vi "GDFreadVariableHeaders.vi"(8 "error in":errorcluster, 11 "GDFv1.x.lvclass in":refnum<class "GDFv1.x.lvclass">) -> (0 "error out":errorcluster, 2 "GDFHeader2 out":T1, 3 "GDFv1.x.lvclass out":refnum<class "GDFv1.x.lvclass">)   [LabVIEW 2016, in "GDF File Reader.lvlib" / "GDFv1.x.lvclass"]
uses:
  GDFv1.x.lvclass
  GdfHeader2.ctl
  GDFv1.x.lvclass/GDFv1.x.ctl
  GDF File Reader.lvlib
panel:
  # "This VI is a part of BCI Design library, http://www.ru-bci.org \nCopyright © 2020, Sotnikov Peter, All rights reserved. License: GNU GPLv3"
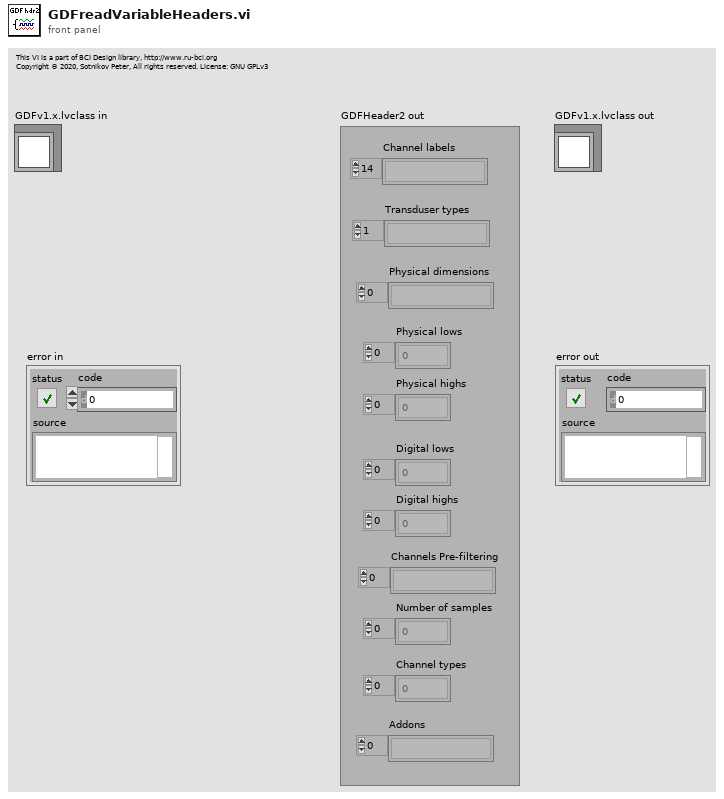
[diagram p1: front panel]
types:
  T1 = typedef "GDF File Reader.lvlib/GdfHeader2.ctl" = cluster{"Channel labels":string[], "Transduser types":string[], "Physical dimensions":string[], "Physical lows":dbl[], "Physical highs":dbl[], "Digital lows":dbl[], "Digital highs":dbl[], "Channels Pre-filtering":string[], "Number of samples":u32[], "Channel types":u32[], "Addons":string[]}
  T2 = typedef "GDF File Reader.lvlib/GdfHeader1.ctl" = cluster{"Version identificator":string, "Patient identificator":string, "Recording identificator":string, "StartDateTime":timestamp, "Header record length":i64, "Equipment Provider":u64, "Laboratory":u64, "Technician":u64, "Number of data records":i64, "Duration of a data record":cluster{"Numerator":u32, "Denominator":u32}, "Number of signals":u32}
  T3 = enum16{"big-endian, network order", "native, host order", "little-endian"}
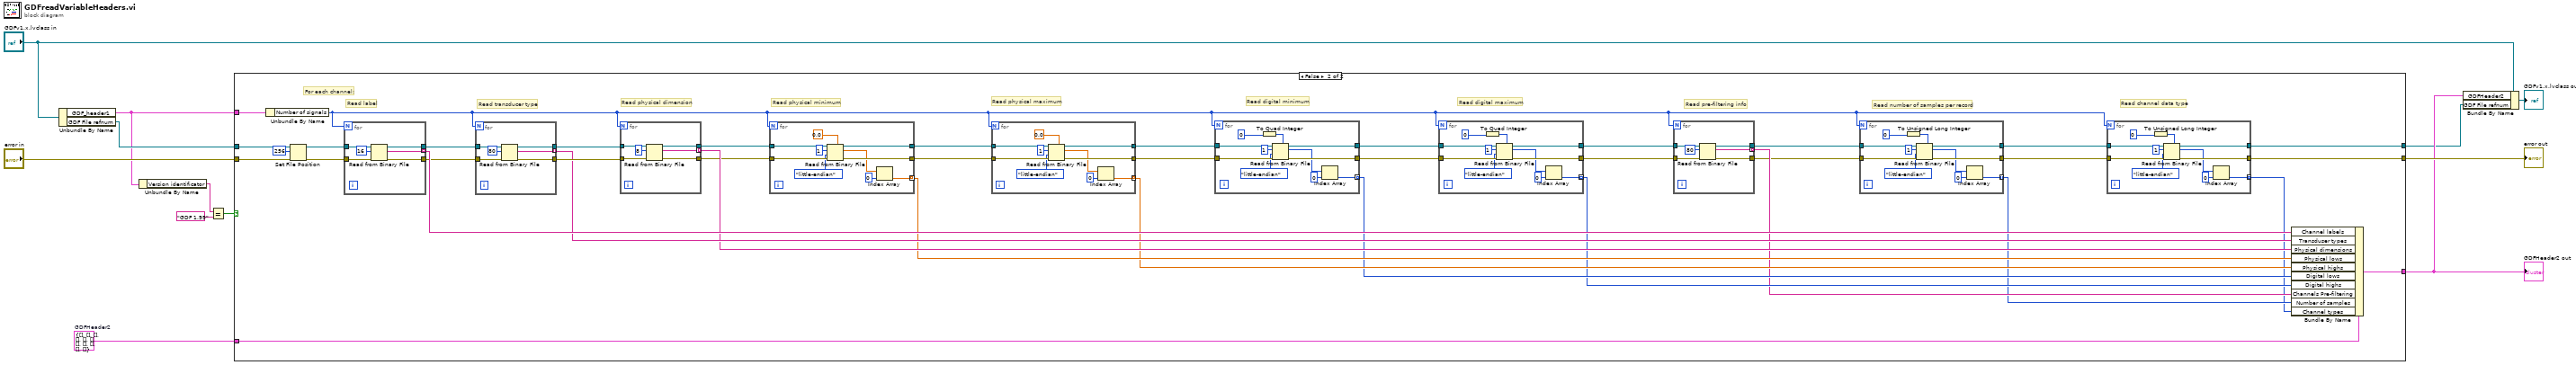
[diagram p0: block diagram]
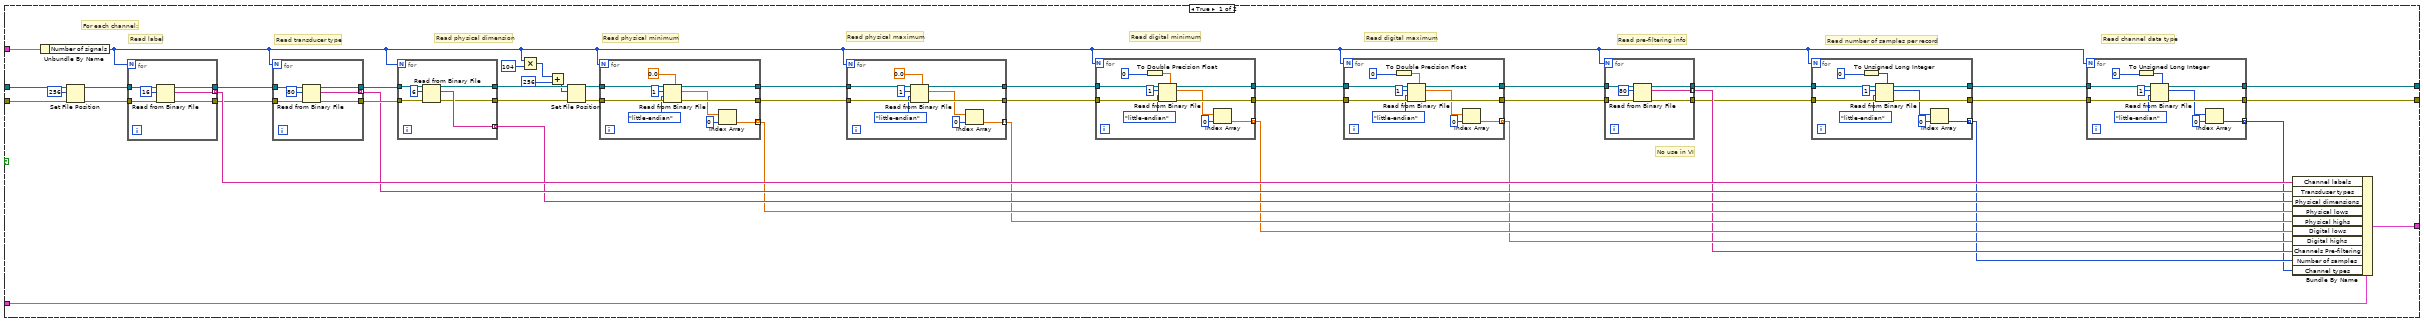
[diagram p2: hidden frame]
diagram:
  w12 = T1 {"Channel labels"=[], "Transduser types"=[], "Physical dimensions"=[], "Physical lows"=[], "Physical highs"=[], "Digital lows"=[], "Digital highs"=[], "Channels Pre-filtering"=[], "Number of samples"=[], "Channel types"=[], "Addons"=[]}  # GDFHeader2
  n1 = Unbundle By Name("GDFv1.x.lvclass in") -> ("GDF_header1"=w4:T2, "GDF File refnum"=w9:refnum<file>)
  n2 = Unbundle By Name(w4) -> ("Version identificator"=w2:string)
  n3 = Equal?(x=w2, y="GDF 1.99") -> (x = y?=w3:bool)
  n4 = case shown="False" w3 {
    tunnel: w12 -> [w57 w184]
    tunnel: "error in" -> [w56 w183]
    tunnel: [w26 w151] -> w10
    tunnel: w9 -> [w25 w149]
    tunnel: w4 -> [w24 w148]
    tunnel: [w23 w147] -> w7
    tunnel: [w22 w146] -> w6
    frame True {
      # "No use in VI"
      # "Read pre-filtering info"
      # "Read channel data type"
      # "Read number of samples per record"
      # "Read digital maximum"
      # "Read digital minimum"
      # "Read physical maximum"
      # "Read physical minimum"
      # "Read physical dimension"
      # "Read transducer type"
      # "Read label"
      # "For each channel:"
      n5 = Unbundle By Name(w24) -> ("Number of signals"=w17:u32)
      n6 = Set File Position(offset (in bytes) (0)=i64 256, refnum=w25, error in=w56) -> (refnum out=w53:refnum<file>, error out=w54:errorcluster)  [unwired: 1 in]
      n7 = for {
        N: w17 -> [_]
        tunnel: w54 -> [w145]
        tunnel: w53 -> [w144]
        tunnel: [w142] -> w50
        tunnel: [w141] -> w51
        tunnel: [w140] -> w52 mode=indexing
        n8 = Read from Binary File(8:w145, 10:16 ("count (1)"), 11:w144) -> (0:w141:errorcluster, 2:w140:string, 3:w142:refnum<file>)  [unwired: 3 in, 1 out]
      }
      n9 = for {
        N: w17 -> [_]
        tunnel: w51 -> [w139]
        tunnel: w50 -> [w138]
        tunnel: [w136] -> w48
        tunnel: [w135] -> w49
        tunnel: [w134] -> w47 mode=indexing
        n10 = Read from Binary File(8:w139, 10:80 ("count (1)"), 11:w138) -> (0:w135:errorcluster, 2:w134:string, 3:w136:refnum<file>)  [unwired: 3 in, 1 out]
      }
      n11 = for {
        N: w17 -> [_]
        tunnel: w49 -> [w133]
        tunnel: w48 -> [w132]
        tunnel: [w128] -> w20
        tunnel: [w129] -> w21
        tunnel: [w130] -> w46 mode=indexing
        n12 = Read from Binary File(8:w133, 10:6 ("count (1)"), 11:w132) -> (0:w129:errorcluster, 2:w130:string, 3:w128:refnum<file>)  [unwired: 3 in, 1 out]
      }
      n13 = Multiply(x=w17, y=u32 104) -> (x*y=w15:u32)
      n14 = Add(x=w15, y=u32 256) -> (x+y=w13:u32)
      n15 = Set File Position(offset (in bytes) (0)=w13, refnum=w20, error in=w21) -> (refnum out=w19:refnum<file>, error out=w18:errorcluster)  [unwired: 1 in]
      n16 = for {
        N: w17 -> [_]
        tunnel: w18 -> [w127]
        tunnel: w19 -> [w126]
        tunnel: [w124] -> w44
        tunnel: [w123] -> w45
        tunnel: [w118] -> w43 mode=indexing
        n17 = Read from Binary File(5:0.0, 8:w127, 9:T3."little-endian" ("byte order (0:big-endian, network order)"), 10:1 ("count (1)"), 11:w126) -> (0:w123:errorcluster, 2:w120:dbl[], 3:w124:refnum<file>)  [unwired: 1 in, 1 out]
        n18 = Index Array(array=w120, index=0) -> (element=w118:dbl)
      }
      n19 = for {
        N: w17 -> [_]
        tunnel: w45 -> [w117]
        tunnel: w44 -> [w116]
        tunnel: [w114] -> w41
        tunnel: [w113] -> w40
        tunnel: [w108] -> w42 mode=indexing
        n20 = Read from Binary File(5:0.0, 8:w117, 9:T3."little-endian" ("byte order (0:big-endian, network order)"), 10:1 ("count (1)"), 11:w116) -> (0:w113:errorcluster, 2:w110:dbl[], 3:w114:refnum<file>)  [unwired: 1 in, 1 out]
        n21 = Index Array(array=w110, index=0) -> (element=w108:dbl)
      }
      n22 = for {
        N: w17 -> [_]
        tunnel: w40 -> [w107]
        tunnel: w41 -> [w106]
        tunnel: [w105] -> w39
        tunnel: [w104] -> w38
        tunnel: [w100] -> w37 mode=indexing
        n23 = To Double Precision Float(number=0 ("count (1)")) -> (double precision float=w97:dbl)
        n24 = Read from Binary File(5:w97, 8:w107, 9:T3."little-endian" ("byte order (0:big-endian, network order)"), 10:1 ("count (1)"), 11:w106) -> (0:w104:errorcluster, 2:w102:dbl[], 3:w105:refnum<file>)  [unwired: 1 in, 1 out]
        n25 = Index Array(array=w102, index=0) -> (element=w100:dbl)
      }
      n26 = for {
        N: w17 -> [_]
        tunnel: w38 -> [w96]
        tunnel: w39 -> [w95]
        tunnel: [w94] -> w34
        tunnel: [w93] -> w35
        tunnel: [w89] -> w36 mode=indexing
        n27 = To Double Precision Float(number=0 ("count (1)")) -> (double precision float=w86:dbl)
        n28 = Read from Binary File(5:w86, 8:w96, 9:T3."little-endian" ("byte order (0:big-endian, network order)"), 10:1 ("count (1)"), 11:w95) -> (0:w93:errorcluster, 2:w91:dbl[], 3:w94:refnum<file>)  [unwired: 1 in, 1 out]
        n29 = Index Array(array=w91, index=0) -> (element=w89:dbl)
      }
      n30 = for {
        N: w17 -> [_]
        tunnel: w35 -> [w85]
        tunnel: w34 -> [w84]
        tunnel: [w82] -> w31
        tunnel: [w81] -> w32
        tunnel: [w80] -> w33 mode=indexing
        n31 = Read from Binary File(8:w85, 10:80 ("count (1)"), 11:w84) -> (0:w81:errorcluster, 2:w80:string, 3:w82:refnum<file>)  [unwired: 3 in, 1 out]
      }
      n32 = for {
        N: w17 -> [_]
        tunnel: w32 -> [w79]
        tunnel: w31 -> [w78]
        tunnel: [w77] -> w29
        tunnel: [w76] -> w30
        tunnel: [w72] -> w28 mode=indexing
        n33 = To Unsigned Long Integer(number=0 ("count (1)")) -> (unsigned 32bit integer=w69:u32)
        n34 = Read from Binary File(5:w69, 8:w79, 9:T3."little-endian" ("byte order (0:big-endian, network order)"), 10:1 ("count (1)"), 11:w78) -> (0:w76:errorcluster, 2:w74:u32[], 3:w77:refnum<file>)  [unwired: 1 in, 1 out]
        n35 = Index Array(array=w74, index=0) -> (element=w72:u32)
      }
      n36 = for {
        N: w17 -> [_]
        tunnel: w30 -> [w68]
        tunnel: w29 -> [w67]
        tunnel: [w66] -> w22
        tunnel: [w65] -> w26
        tunnel: [w61] -> w27 mode=indexing
        n37 = To Unsigned Long Integer(number=0 ("count (1)")) -> (unsigned 32bit integer=w58:u32)
        n38 = Read from Binary File(5:w58, 8:w68, 9:T3."little-endian" ("byte order (0:big-endian, network order)"), 10:1 ("count (1)"), 11:w67) -> (0:w65:errorcluster, 2:w63:u32[], 3:w66:refnum<file>)  [unwired: 1 in, 1 out]
        n39 = Index Array(array=w63, index=0) -> (element=w61:u32)
      }
      n40 = Bundle By Name(cluster=w57, "Channel labels"=w52, "Transduser types"=w47, "Physical dimensions"=w46, "Physical lows"=w43, "Physical highs"=w42, "Digital lows"=w37, "Digital highs"=w36, "Channels Pre-filtering"=w33, "Number of samples"=w28, "Channel types"=w27) -> (w23:T1)
    }
    frame False {
      # "Read pre-filtering info"
      # "Read channel data type"
      # "Read number of samples per record"
      # "Read digital maximum"
      # "Read digital minimum"
      # "Read physical maximum"
      # "Read physical minimum"
      # "Read physical dimension"
      # "Read transducer type"
      # "Read label"
      # "For each channel:"
      n41 = Unbundle By Name(w148) -> ("Number of signals"=w150:u32)
      n42 = Set File Position(offset (in bytes) (0)=i64 256, refnum=w149, error in=w183) -> (refnum out=w180:refnum<file>, error out=w181:errorcluster)  [unwired: 1 in]
      n43 = for {
        N: w150 -> [_]
        tunnel: w181 -> [w272]
        tunnel: w180 -> [w271]
        tunnel: [w269] -> w177
        tunnel: [w268] -> w178
        tunnel: [w267] -> w179 mode=indexing
        n44 = Read from Binary File(8:w272, 10:16 ("count (1)"), 11:w271) -> (0:w268:errorcluster, 2:w267:string, 3:w269:refnum<file>)  [unwired: 3 in, 1 out]
      }
      n45 = for {
        N: w150 -> [_]
        tunnel: w178 -> [w266]
        tunnel: w177 -> [w265]
        tunnel: [w263] -> w175
        tunnel: [w262] -> w176
        tunnel: [w261] -> w174 mode=indexing
        n46 = Read from Binary File(8:w266, 10:80 ("count (1)"), 11:w265) -> (0:w262:errorcluster, 2:w261:string, 3:w263:refnum<file>)  [unwired: 3 in, 1 out]
      }
      n47 = for {
        N: w150 -> [_]
        tunnel: w176 -> [w260]
        tunnel: w175 -> [w259]
        tunnel: [w257] -> w172
        tunnel: [w256] -> w171
        tunnel: [w255] -> w173 mode=indexing
        n48 = Read from Binary File(8:w260, 10:8 ("count (1)"), 11:w259) -> (0:w256:errorcluster, 2:w255:string, 3:w257:refnum<file>)  [unwired: 3 in, 1 out]
      }
      n49 = for {
        N: w150 -> [_]
        tunnel: w171 -> [w254]
        tunnel: w172 -> [w253]
        tunnel: [w251] -> w169
        tunnel: [w250] -> w170
        tunnel: [w245] -> w168 mode=indexing
        n50 = Read from Binary File(5:0.0, 8:w254, 9:T3."little-endian" ("byte order (0:big-endian, network order)"), 10:1 ("count (1)"), 11:w253) -> (0:w250:errorcluster, 2:w247:dbl[], 3:w251:refnum<file>)  [unwired: 1 in, 1 out]
        n51 = Index Array(array=w247, index=0) -> (element=w245:dbl)
      }
      n52 = for {
        N: w150 -> [_]
        tunnel: w170 -> [w244]
        tunnel: w169 -> [w243]
        tunnel: [w241] -> w166
        tunnel: [w240] -> w165
        tunnel: [w235] -> w167 mode=indexing
        n53 = Read from Binary File(5:0.0, 8:w244, 9:T3."little-endian" ("byte order (0:big-endian, network order)"), 10:1 ("count (1)"), 11:w243) -> (0:w240:errorcluster, 2:w237:dbl[], 3:w241:refnum<file>)  [unwired: 1 in, 1 out]
        n54 = Index Array(array=w237, index=0) -> (element=w235:dbl)
      }
      n55 = for {
        N: w150 -> [_]
        tunnel: w165 -> [w234]
        tunnel: w166 -> [w233]
        tunnel: [w232] -> w164
        tunnel: [w231] -> w163
        tunnel: [w227] -> w162 mode=indexing
        n56 = To Quad Integer(1:0 ("count (1)")) -> (0:w224:i64)
        n57 = Read from Binary File(5:w224, 8:w234, 9:T3."little-endian" ("byte order (0:big-endian, network order)"), 10:1 ("count (1)"), 11:w233) -> (0:w231:errorcluster, 2:w229:i64[], 3:w232:refnum<file>)  [unwired: 1 in, 1 out]
        n58 = Index Array(array=w229, index=0) -> (element=w227:i64)
      }
      n59 = for {
        N: w150 -> [_]
        tunnel: w163 -> [w223]
        tunnel: w164 -> [w222]
        tunnel: [w221] -> w159
        tunnel: [w220] -> w160
        tunnel: [w216] -> w161 mode=indexing
        n60 = To Quad Integer(1:0 ("count (1)")) -> (0:w213:i64)
        n61 = Read from Binary File(5:w213, 8:w223, 9:T3."little-endian" ("byte order (0:big-endian, network order)"), 10:1 ("count (1)"), 11:w222) -> (0:w220:errorcluster, 2:w218:i64[], 3:w221:refnum<file>)  [unwired: 1 in, 1 out]
        n62 = Index Array(array=w218, index=0) -> (element=w216:i64)
      }
      n63 = for {
        N: w150 -> [_]
        tunnel: w160 -> [w212]
        tunnel: w159 -> [w211]
        tunnel: [w209] -> w156
        tunnel: [w208] -> w157
        tunnel: [w207] -> w158 mode=indexing
        n64 = Read from Binary File(8:w212, 10:80 ("count (1)"), 11:w211) -> (0:w208:errorcluster, 2:w207:string, 3:w209:refnum<file>)  [unwired: 3 in, 1 out]
      }
      n65 = for {
        N: w150 -> [_]
        tunnel: w157 -> [w206]
        tunnel: w156 -> [w205]
        tunnel: [w204] -> w154
        tunnel: [w203] -> w155
        tunnel: [w199] -> w153 mode=indexing
        n66 = To Unsigned Long Integer(number=0 ("count (1)")) -> (unsigned 32bit integer=w196:u32)
        n67 = Read from Binary File(5:w196, 8:w206, 9:T3."little-endian" ("byte order (0:big-endian, network order)"), 10:1 ("count (1)"), 11:w205) -> (0:w203:errorcluster, 2:w201:u32[], 3:w204:refnum<file>)  [unwired: 1 in, 1 out]
        n68 = Index Array(array=w201, index=0) -> (element=w199:u32)
      }
      n69 = for {
        N: w150 -> [_]
        tunnel: w155 -> [w195]
        tunnel: w154 -> [w194]
        tunnel: [w193] -> w146
        tunnel: [w192] -> w151
        tunnel: [w188] -> w152 mode=indexing
        n70 = To Unsigned Long Integer(number=0 ("count (1)")) -> (unsigned 32bit integer=w185:u32)
        n71 = Read from Binary File(5:w185, 8:w195, 9:T3."little-endian" ("byte order (0:big-endian, network order)"), 10:1 ("count (1)"), 11:w194) -> (0:w192:errorcluster, 2:w190:u32[], 3:w193:refnum<file>)  [unwired: 1 in, 1 out]
        n72 = Index Array(array=w190, index=0) -> (element=w188:u32)
      }
      n73 = Bundle By Name(cluster=w184, "Channel labels"=w179, "Transduser types"=w174, "Physical dimensions"=w173, "Physical lows"=w168, "Physical highs"=w167, "Digital lows"=w162, "Digital highs"=w161, "Channels Pre-filtering"=w158, "Number of samples"=w153, "Channel types"=w152) -> (w147:T1)
    }
  }
  "GDFHeader2 out" <- w7
  "error out" <- w10
  n74 = Bundle By Name(cluster="GDFv1.x.lvclass in", "GDFHeader2"=w7, "GDF File refnum"=w6) -> (→"GDFv1.x.lvclass out":refnum<class "GDFv1.x.lvclass">)
